vi "_Update Method Parameters.vi"(9 "Parameter Value":dbl[](array[numeric]), 10 "Ch#":u8[](array[numeric]), 11 "Method File":path) -> (0 "error out":errorcluster)   [LabVIEW 2012]
uses:
  Type/_File Type.ctl
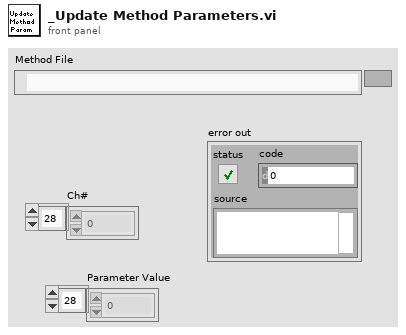
[diagram p1: front panel]
types:
  T1 = typedef "_File Type.ctl" = enum16{"Configuration", "Old Configuration", "Calibration", "Resolution", "Diagnostic Method", "Old Method", "Acq Method", "Samp List"}
  T2 = typedef "_GUI Method.ctl" = cluster{"Lenses":T3[], "Mass Ranges":T4[], "Acquire":bool, "MCA":bool, "Q1DC EN":bool, "Q1 POL":bool, "Q3 POL":bool, "Q1 RF  EN":bool, "Averaging":bool, "Log Scale":bool, "CPS":bool, "Unit":bool, "Data Path":path, "Run Mode":T7, "Fixed Mass (amu)":dbl, "Q3DC EN":bool, "Q3 RF  EN":bool, "Negative":bool}
  T3 = typedef "_Lens Property.ctl" = cluster{"Scan Type":u8, "Scans":i32, "Time 1":dbl, "Time 2":dbl, "Value 1":dbl, "Value 2":dbl, "Step Size":dbl}
  T4 = typedef "_Mass Range Property.ctl" = cluster{"Start":dbl, "Stop":dbl, "Step Size":dbl, "Steps":i32, "Dwell":dbl, "Parameters":T5[], "Res":T6}
  T5 = typedef "_Mass Range Parameters.ctl" = cluster{"Name":string, "Ch#":u8, "StartV":dbl, "StopV":dbl, "StepV":dbl, "Index":u8}
  T6 = typedef "_RT Res Type.ctl" = u16
  T7 = typedef "_Run Mode.ctl" = enum16{"MRM (Q1/Q2)", "Q1 Scan", "Q1 SRM", "Q2 Scan", "Q2 SRM", "Product Scan", "Precursor Scan", "Neutral Loss", "Neutral Gain"}
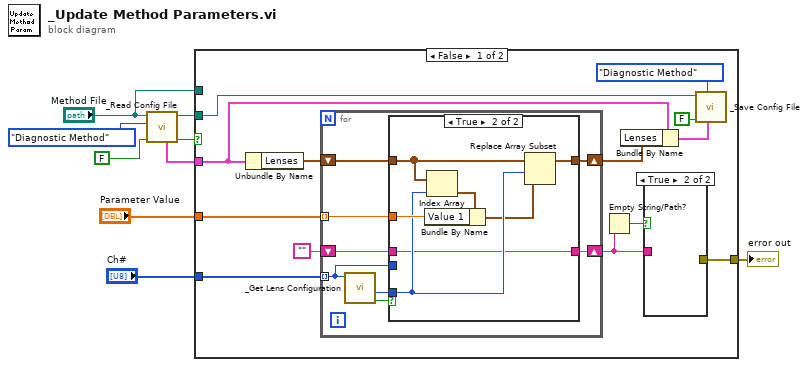
[diagram p0: block diagram]
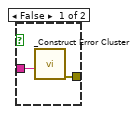
[diagram p2: hidden frame]
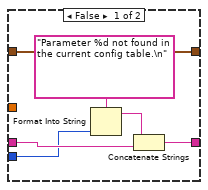
[diagram p3: hidden frame]
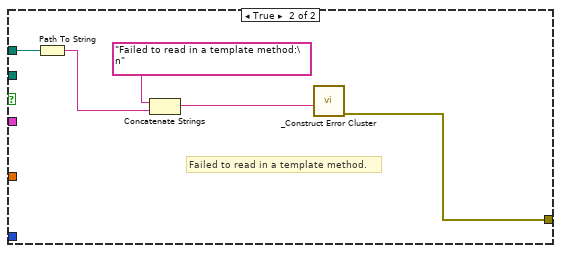
[diagram p4: hidden frame]
diagram:
  n1 = call "_Read Config File.vi"("advisory dialog? (display:T)"=FALSE, "File Type (config)"=_File_Type."Diagnostic Method", "start path  (Not A Path)"="Method File") -> ("error"=w7:bool, "new file path"=w4:path, "GUI Method"=w6:T2)  [unwired: 6 out]
  n2 = case shown="False" w7 {
    tunnel: w6 -> [w22 _]
    tunnel: "Ch#" -> [w17 _]
    tunnel: w4 -> [w20 _]
    tunnel: "Parameter Value" -> [w18 _]
    tunnel: "Method File" -> [_ w49]
    tunnel: [w11 w46] -> w1
    frame False {
      n3 = Unbundle By Name(w22) -> ("Lenses"=w16:T3[])
      n4 = for {
        tunnel: w18 -> [w29] mode=indexing
        tunnel: w17 -> [w25] mode=indexing
        shift-right: [w26] -> w12
        shift-left: "" -> [w27]
        shift-right: [w28] -> w15
        shift-left: w16 -> [w30]
        n5 = call "_Get Lens Configuration.vi"("Channel #"=w25) -> ("Found"=w32:bool, "Config Row#"=w31:i32)  [unwired: 4 in, 1 out]
        n6 = case shown="True" w32 {
          tunnel: w31 -> [_ w42]
          tunnel: w30 -> [w38 w43]
          tunnel: w29 -> [_ w44]
          tunnel: [w38 w40] -> w28
          tunnel: w27 -> [w37 w39]
          tunnel: [w36 w39] -> w26
          tunnel: w25 -> [w34 _]
          frame False {
            n7 = Format Into String(format string="Parameter %d not found in the current config table.\n", w34) -> (resulting string=w33:string)  [unwired: 2 in, 1 out]
            n8 = Concatenate Strings(w33, w37) -> (w36:string)
          }
          frame True {
            n9 = Index Array(array=w43, index=w42) -> (element=w45:T3)
            n10 = Bundle By Name(cluster=w45, "Value 1"=w44) -> (w41:T3)
            n11 = Replace Array Subset(array=w43, new element=w41, index=w42) -> (w40:T3[])
          }
        }
      }
      n12 = Empty String/Path?(string/path=w12) -> (empty?=w13:bool)
      n13 = Bundle By Name(cluster=w22, "Lenses"=w15) -> (w19:T2)
      n14 = case shown="True" w13 {
        tunnel: w12 -> [w24 _]
        tunnel: [w23 _] -> w11
        frame False {
          n15 = call "_Construct Error Cluster.vi"("reason"=w24) -> ("error out"=w23:errorcluster)  [unwired: 6 in]
        }
        frame True {
        }
      }
      n16 = call "_Save Config File.vi"("GUI Method"=w19, "File Type (config)"=_File_Type."Diagnostic Method", "advisory dialog? (display:T)"=FALSE, "start path  (Not A Path)"=w20) -> ()  [unwired: 4 in, 4 out]
    }
    frame True {
      # "Failed to read in a template method."
      n17 = Path To String(path=w49) -> (string=w48:string)
      n18 = Concatenate Strings("Failed to read in a template method:\n", w48) -> (w47:string)
      n19 = call "_Construct Error Cluster.vi"("reason"=w47) -> ("error out"=w46:errorcluster)  [unwired: 6 in]
    }
  }
  "error out" <- w1
